vi "Clear Task.vi"(8 "error in":errorcluster, 11 "NI Digital Input in":refnum<class "NI Digital Input.lvclass">) -> (0 "error out":errorcluster, 3 "NI Digital Input out":refnum<class "NI Digital Input.lvclass">)   [LabVIEW 2023, in "HardwareAbstractionLayer_LVOOP.lvlib" / "NI Digital Input.lvclass"]
doc: "This VI DAXmx Clear Task"
uses:
  NI Digital Input.lvclass
  NI Digital Input.lvclass/NI Digital Input.ctl
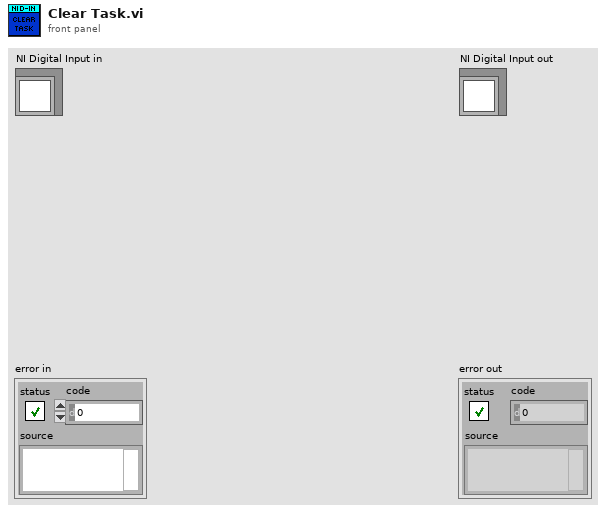
[diagram p1: front panel]
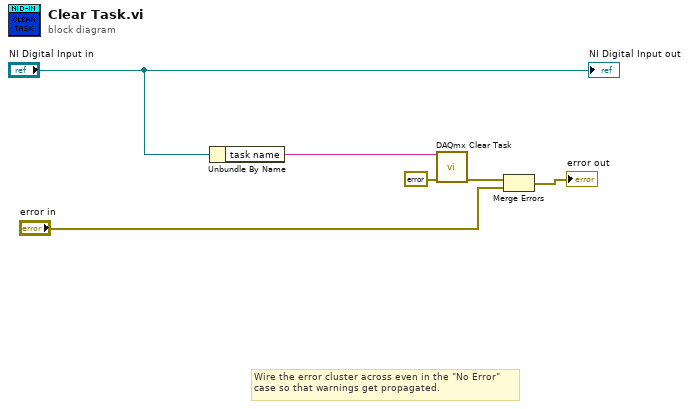
[diagram p0: block diagram]
diagram:
  # "Wire the error cluster across even in the \"No Error\"\ncase so that warnings get propagated."
  n1 = Unbundle By Name("NI Digital Input in") -> ("task name"=w4:string)
  n2 = call <vilib>:"DAQmx Clear Task.vi"("task in"=w4, "error in"=errorcluster {"status"=FALSE, "code"=0, "source"=""}) -> ("error out"=w6:errorcluster)  [unwired: 13 in]
  n3 = Merge Errors(w6, "error in") -> (→"error out":errorcluster)
  "NI Digital Input out" <- "NI Digital Input in"
